vi "IsBool.vi"(4 "Value String in":string) -> (0 "IsBool":bool, 2 "Bool Value":bool)   [LabVIEW 2019]
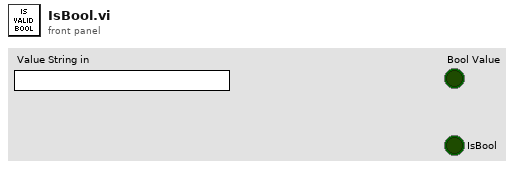
[diagram p1: front panel]
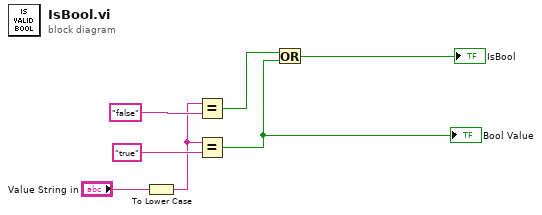
[diagram p0: block diagram]
diagram:
  n1 = To Lower Case(string="Value String in") -> (all lower case string=w4:string)
  n2 = Equal?(x=w4, y="false") -> (x = y?=w3:bool)
  n3 = Equal?(x=w4, y="true") -> (x = y?=w1:bool)
  "Bool Value" <- w1
  n4 = Or(x=w3, y=w1) -> (x .or. y?=→"IsBool":bool)
